vi "Supply_SetVolts.vi"(8 "error in (no error)":errorcluster, 9 "Command string":string, 10 "Volts IN [V]":dbl, 11 "KE2657A in":refnum<class "KE2657A.lvclass">) -> (0 "error out":errorcluster, 2 "Compliance exceeded?":bool, 3 "KE2657A out":refnum<class "KE2657A.lvclass">)   [LabVIEW 2018, in "KE2657A.lvclass"]
uses:
  KE2657A.lvclass
  SupplyControl.lvclass
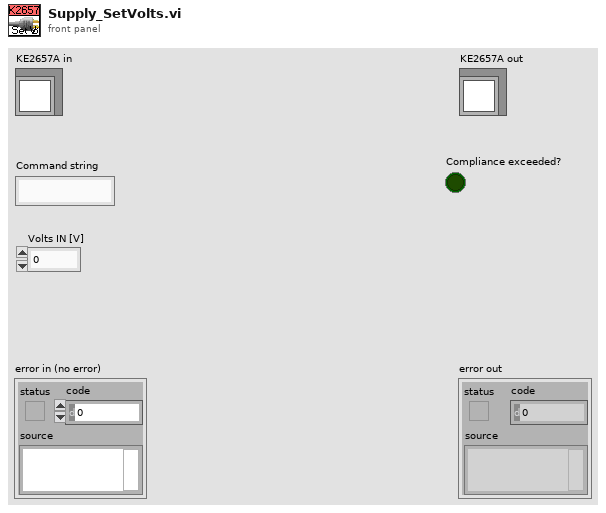
[diagram p1: front panel]
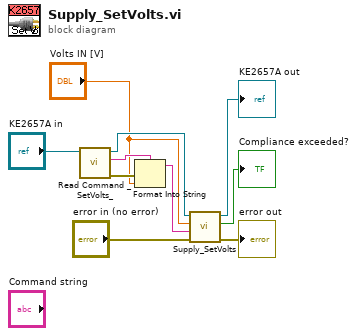
[diagram p0: block diagram]
diagram:
  n1 = call-dynamic "Read Command _SetVolts_.vi"("SupplyControl in"="KE2657A in") -> ("error out"=w4:errorcluster, "Command \"SetVolts\""=w5:string, "SupplyControl out"=w3:refnum<class "KE2657A.lvclass">)  [unwired: 8 in]
  n2 = Format Into String(format string=w5, error in=w4, "Volts IN [V]") -> (resulting string=w2:string)  [unwired: 1 in, 1 out]
  n3 = call-parent "Supply_SetVolts.vi"("error in (no error)"="error in (no error)", "Command string"=w2, "Volts IN [V]"="Volts IN [V]", "SupplyControl in"=w3) -> ("error out"=→"error out":errorcluster, "Compliance exceeded?"=→"Compliance exceeded?":bool, "SupplyControl out"=→"KE2657A out":refnum<class "KE2657A.lvclass">)  [unwired: 5 in]
